vi "Automation.vi"() -> ()   [LabVIEW 2018]
uses:
  <vilib>/Utility/error.llb/DialogType.ctl
  cb6d7afe-07a1-4717-8708-8a88368bf63c.vi
panel:
  in  "Ref Level Auto":bool=TRUE
  out "Min":dbl
  out "Sec":dbl
  out "H":dbl
  in  "Stop Button":bool
  out "P x Lambda Graph":cluster{dbl[], dbl[]}(graph)
  out "Corrente Atual (mA)":dbl
  out "P x I Graph":cluster{dbl[], dbl[]}(graph)
  in  "Start Button":bool
  in  "Cluster de Dados de Entrada":T1={"Corrente Inicial (mA)"=30.0, "Limite de Temperatura"=27.0, "Temperatura"=25.0, "Corrente Limite (mA)"=300, "Centralizar pico (nm)"=1557.0, "Valor de Span (nm)"=20.0, "Passo (mA)"=10.0, "Corrente Final (mA)"=650.0, "Resolucao"=enum."High"} {"Corrente Final (mA)" min=0.0 step=1.0; "Passo (mA)" min=1.0 step=1.0; "Valor de Span (nm)" min=0.1 max=1400.0 format="%.2f"; "Centralizar pico (nm)" format="%.2f"; "Temperatura" min=-100.0 max=199.9 step=0.1; "Limite de Temperatura" min=-100.0 max=199.9 step=0.1; "Corrente Inicial (mA)" min=0.0 step=1.0}
  out "XY Graph":T2(graph)
  in  "Pasta Destino":path=path "d:/Users/Stinky/Documents/11.04.2019/aquisicao14_HR_4mA_151_500"
  in  "GPIB Analisador de Espectros":refnum<visa-resource-name>="Advantest_Spectrometer_82357A"
  in  "GPIB Controlador Laser Diodo":refnum<visa-resource-name>="DiodeLaserController__82357A"
  in  "error in (no error)":errorcluster
  out "error out":errorcluster
  # "Tempo Gasto"
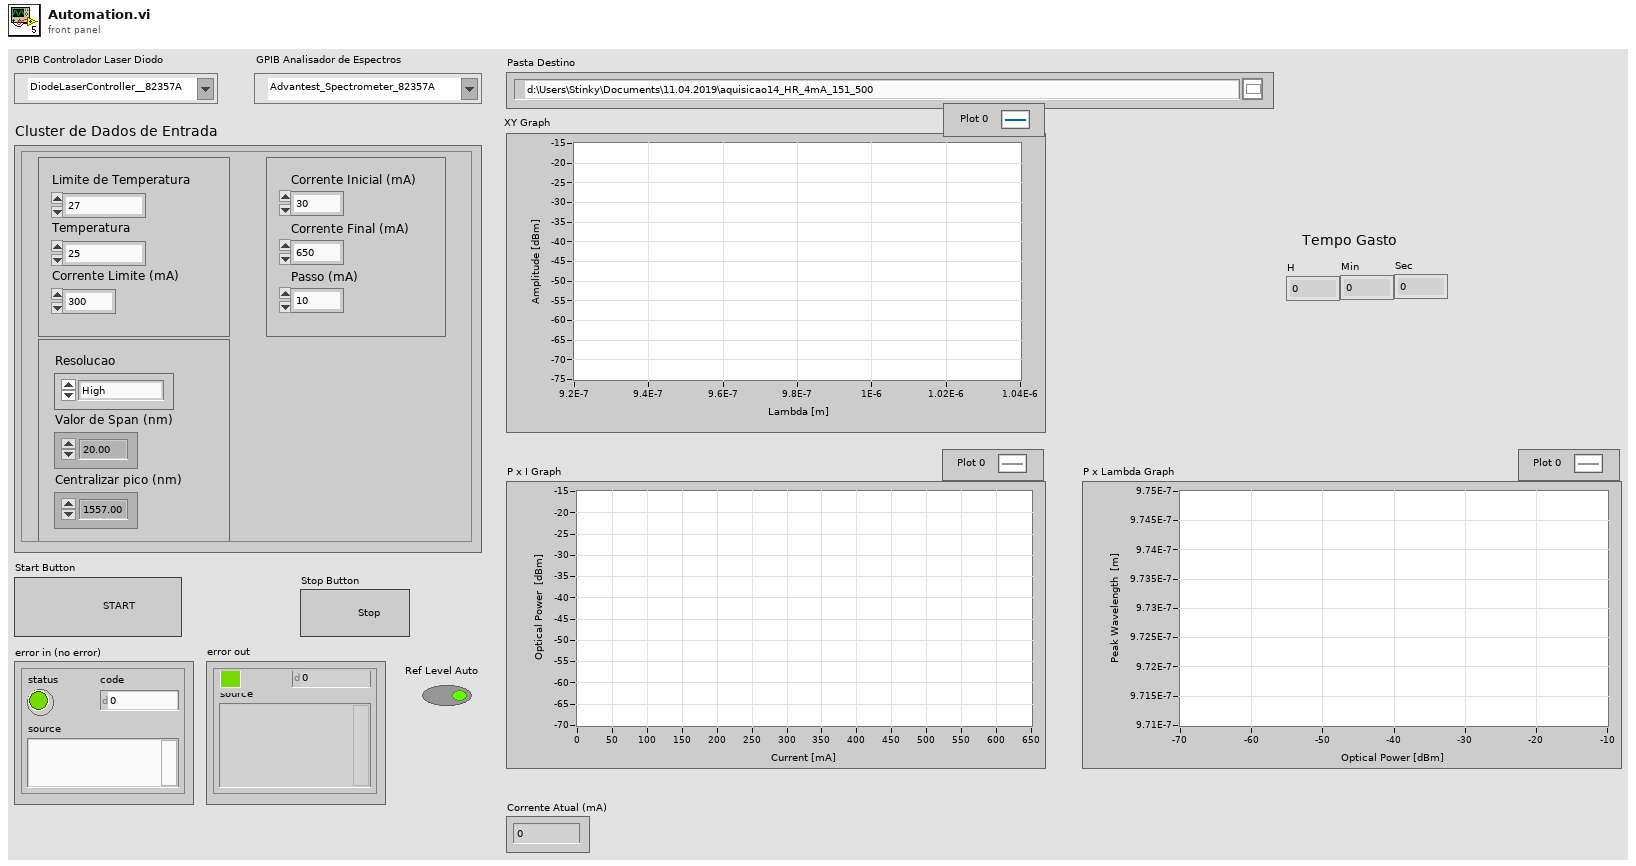
[diagram p1: front panel]
types:
  T1 = cluster{"Corrente Inicial (mA)":dbl, "Limite de Temperatura":dbl, "Temperatura":dbl, "Corrente Limite (mA)":i32, "Centralizar pico (nm)":dbl, "Valor de Span (nm)":dbl, "Passo (mA)":dbl, "Corrente Final (mA)":dbl, "Resolucao":enum16{"Normal", "High"}}
  T2 = cluster{"Wavelike Data":dbl[], "Wavelike Data":dbl[]}
  T3 = typedef "DialogType.ctl" = u16
  T4 = cluster{"Limite de Temperatura":dbl, "Temperatura":dbl, "Corrente Inicial (mA)":dbl, "Corrente Limite (mA)":i32, "Resolucao":enum16{"Normal", "High"}, "Centralizar pico (nm)":dbl, "Valor de Span (nm)":dbl}
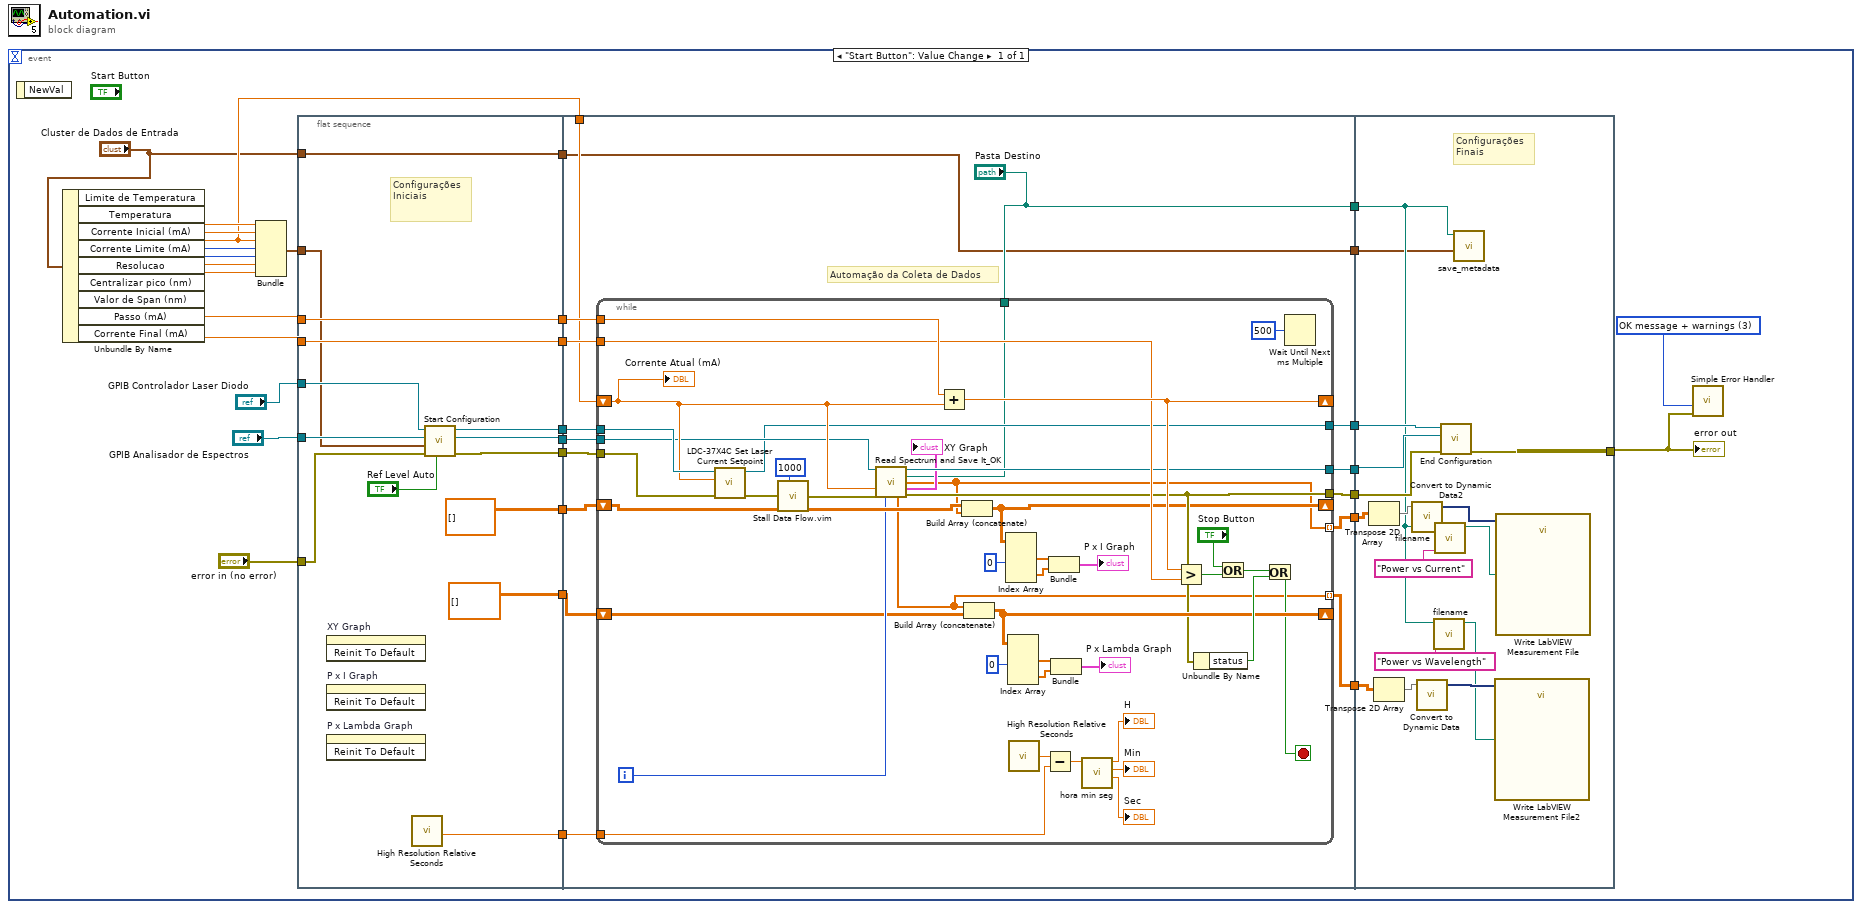
[diagram p0: block diagram]
diagram:
  n1 = event shown="[0] \"Start Button\": Value Change" {
    selector: _ -> [_]
    dyn-events: _ -> [_]
    timeout: _ -> [_]
    event "Start Button": Value Change {
      w9 = T3 3 items=["no dialog", "OK message", "continue or stop message", "OK message + warnings", "continue/stop + warnings"] ("type of dialog (OK msg:1)")
      n2 = event-data() -> ()  [unwired: 1 in, 1 out]
      n3 = Unbundle By Name("Cluster de Dados de Entrada") -> ("Limite de Temperatura"=w23:dbl, "Temperatura"=w22:dbl, "Corrente Inicial (mA)"=w14:dbl, "Corrente Limite (mA)"=w21:i32, "Resolucao"=w20:enum16{"Normal", "High"}, "Centralizar pico (nm)"=w19:dbl, "Valor de Span (nm)"=w17:dbl, "Passo (mA)"=w16:dbl, "Corrente Final (mA)"=w15:dbl)
      n4 = Bundle("Limite de Temperatura"=w23, "Temperatura"=w22, "Corrente Inicial (mA)"=w14, "Corrente Limite (mA)"=w21, "Resolucao"=w20, "Centralizar pico (nm)"=w19, "Valor de Span (nm)"=w17) -> (w18:T4)  [unwired: 1 in]
      n5 = flat-sequence {
        tunnel: "error in (no error)" -> [w38]
        tunnel: [w46] -> w32
        tunnel: [w45] -> w31
        tunnel: "GPIB Controlador Laser Diodo" -> [w44]
        tunnel: "GPIB Analisador de Espectros" -> [w43]
        tunnel: [w42] -> w30
        tunnel: [w41] -> w29
        tunnel: w16 -> [w41]
        tunnel: w15 -> [w40]
        tunnel: [w40] -> w28
        tunnel: w18 -> [w35]
        tunnel: [dbl[][] []] -> w13
        tunnel: [dbl[][] []] -> w8
        tunnel: [w36] -> w7
        tunnel: [w34] -> w3
        tunnel: "Cluster de Dados de Entrada" -> [w34]
        tunnel: w32 -> [w62]
        tunnel: w31 -> [w61]
        tunnel: w30 -> [w60]
        tunnel: [w59] -> w27
        tunnel: w29 -> [w58]
        tunnel: w28 -> [w57]
        tunnel: w14 -> [w56]
        tunnel: w13 -> [w55]
        tunnel: [w54] -> w12
        tunnel: [w53] -> w11
        tunnel: w8 -> [w52]
        tunnel: w7 -> [w51]
        tunnel: ["Pasta Destino"] -> w6
        tunnel: [w49] -> w5
        tunnel: [w48] -> w4
        tunnel: w3 -> [w47]
        tunnel: [w47] -> w2
        tunnel: [w120] -> w10
        tunnel: w27 -> [w119]
        tunnel: w12 -> [w118]
        tunnel: w11 -> [w117]
        tunnel: w6 -> [w106]
        tunnel: w5 -> [w108]
        tunnel: w4 -> [w110]
        tunnel: w2 -> [w105]
        frame #0 {
          # "Configurações\nIniciais"
          n6 = invoke on="XY Graph" class="XYGraph (strict)" method="Reinit To Default"() -> ()  [unwired: 3 in, 3 out]
          n7 = invoke on="P x I Graph" class="XYGraph (strict)" method="Reinit To Default"() -> ()  [unwired: 3 in, 3 out]
          n8 = invoke on="P x Lambda Graph" class="XYGraph (strict)" method="Reinit To Default"() -> ()  [unwired: 3 in, 3 out]
          n9 = call <vilib>:"High Resolution Relative Seconds.vi"() -> ("relative seconds"=w36:dbl)
          n10 = call "Start Configuration.vi"("Ref Lvl Auto"="Ref Level Auto", "error in (no error)"=w38, "Cluster de Dados"=w35, "GPIB Espectrometro"=w43, "GPIB Controlador Laser Diodo"=w44) -> ("error out"=w46:errorcluster, "Spectrometer out"=w42:refnum<visa-resource-name>, "Controller out"=w45:refnum<visa-resource-name>)  [unwired: 4 in]
        }
        frame #1 {
          # "Automação da Coleta de Dados"
          n11 = while {
            shift-right: [w98] -> _
            shift-left: w56 -> [w99]
            tunnel: w62 -> [w91]
            tunnel: w61 -> [w104]
            tunnel: w60 -> [w97]
            tunnel: [w94] -> w59
            tunnel: w58 -> [w96]
            tunnel: w57 -> [w95]
            shift-right: [w65] -> _
            shift-left: w55 -> [w90]
            tunnel: [w78] -> w54
            tunnel: [w85] -> w53
            shift-right: [w79] -> _
            shift-left: w52 -> [w80]
            tunnel: w51 -> [w74]
            tunnel: "Pasta Destino" -> [w66]
            tunnel: [w64] -> w49 mode=indexing
            tunnel: [w63] -> w48 mode=indexing
            i -> [w86]
            stop <- w76 stop-if-true
            n12 = call "LDC-37X4C Set Laser Current Setpoint.vi"("error in (no error)"=w91, "Current"=w99, "VISA resource name"=w104) -> ("error out"=w102:errorcluster, "VISA resource name out"=w94:refnum<visa-resource-name>)  [unwired: 7 in]
            n13 = call "Stall Data Flow.vim"("value in"=w102, "milliseconds to wait"=u32 1000) -> ("value out"=w100:errorcluster)  [unwired: 1 out]
            n14 = call "Read Spectrum and Save It_OK.vi"("VISA Session"=w97, "Pasta Destino DESTA aquisicao"=w66, "Corrente Atual (mA)"=w99, "Error In"=w100, "Iteracao"=w86) -> ("Copy VISA Session"=w85:refnum<visa-resource-name>, "PxI"=w63:dbl[], "XY Graph"=→"XY Graph":T2, "PxLambda"=w64:dbl[], "Error Out"=w78:errorcluster)  [unwired: 4 in, 2 out]
            n15 = Add(x=w96, y=w99) -> (x+y=w98:dbl)
            n16 = Build Array (concatenate)(w90, w63) -> (w65:dbl[][])
            n17 = Build Array (concatenate)(w64, w80) -> (w79:dbl[][])
            n18 = Index Array(array=w65, index (col) #1=0 ("disabled index (col)")) -> (element #1=w88:dbl[], element #2=w87:dbl[])  [unwired: 3 in]
            n19 = Index Array(array=w79, index (col) #1=0 ("disabled index (col)")) -> (element #1=w82:dbl[], element #2=w81:dbl[])  [unwired: 3 in]
            n20 = call <vilib>:"High Resolution Relative Seconds.vi"() -> ("relative seconds"=w75:dbl)
            n21 = Subtract(x=w75, y=w74) -> (x-y=w73:dbl)
            n22 = Bundle(w88, w87) -> (→"P x I Graph":cluster{dbl[], dbl[]})  [unwired: 1 in]
            n23 = Bundle(w82, w81) -> (→"P x Lambda Graph":cluster{dbl[], dbl[]})  [unwired: 1 in]
            n24 = call "hora min seg.vi"("Total time in seconds"=w73) -> ("Sec"=→"Sec":dbl, "Min"=→"Min":dbl, "H"=→"H":dbl)  [unwired: 8 in]
            n25 = Greater?(x=w98, y=w95) -> (0:w101:bool)
            n26 = Unbundle By Name(w78) -> ("status"=w92:bool)
            n27 = Or(x="Stop Button", y=w101) -> (x .or. y?=w93:bool)
            n28 = Or(x=w93, y=w92) -> (x .or. y?=w76:bool)
            n29 = Wait Until Next ms Multiple(millisecond multiple=u32 500) -> ()  [unwired: 1 out]
            "Corrente Atual (mA)" <- w99
          }
        }
        frame #2 {
          # "Configurações\nFinais"
          n30 = Transpose 2D Array(2D array=w110) -> (transposed array=w109:dbl[][])
          n31 = Transpose 2D Array(2D array=w108) -> (transposed array=w107:dbl[][])
          n32 = call "Convert to Dynamic Data2"("2D Array"=w109) -> ("Dynamic Data Type"=w113:dynamicdata)  [unwired: 3 in]
          n33 = call "Convert to Dynamic Data"("2D Array"=w107) -> ("Dynamic Data Type"=w114:dynamicdata)  [unwired: 3 in]
          n34 = call "filename.vi"("Filename"="Power vs Wavelength", "Pasta Destino"=w106) -> ("filename output"=w111:path)  [unwired: 9 in]
          n35 = call "filename.vi"("Filename"="Power vs Current", "Pasta Destino"=w106) -> ("filename output"=w112:path)  [unwired: 9 in]
          n36 = call "End Configuration.vi"("error in (no error)"=w118, "GPIB Espectrometro"=w117, "GPIB Controlador Laser Diodo"=w119) -> ("error out"=w120:errorcluster)  [unwired: 8 in]
          n37 = call "save_metadata.vi"("Cluster de Dados de Entrada"=w105, "Pasta Destino"=w106) -> ()  [unwired: 10 in]
          n38 = call "Write LabVIEW Measurement File2"("Signals"=w114, "Filename"=w111) -> ()  [unwired: 15 in, 3 out]
          n39 = call "Write LabVIEW Measurement File"("Signals"=w113, "Filename"=w112) -> ()  [unwired: 15 in, 3 out]
        }
      }
      n40 = call <vilib>:"Simple Error Handler.vi"("type of dialog (OK msg:1)"=w9, "error in (no error)"=w10) -> ()  [unwired: 3 in, 5 out]
      "error out" <- w10
    }
  }
